vi "Format Error To Log Entry.vi"(6 "Error Call Chain":string[](array[string]), 7 "Event Level":T1, 8 "Error To Log":errorcluster, 9 "Event Time":timestamp, 10 "Error SourceID":string, 11 "Application Logger In":refnum<class "Application Logger.lvclass">) -> (2 "Log Packet":T2, 3 "Application Logger out":refnum<class "Application Logger.lvclass">)   [LabVIEW 2020, in "Composed Log.lvlib" / "Application Logger.lvclass"]
uses:
  <vilib>/gpm_packages/@cs/event-logger/Source/Composed Log/Application Logger/Application Logger.lvclass
  <vilib>/gpm_packages/@cs/event-logger/Source/Composed Log/Types/Log Packet.ctl
  <vilib>/gpm_packages/@cs/event-logger/Source/Composed Log/Types/Log Level.ctl
  <vilib>/gpm_packages/@cs/event-logger/Source/Composed Log/IErrorFormat/IErrorFormat.lvclass
  <vilib>/gpm_packages/@cs/event-logger/Source/Composed Log/Application Logger/Application Logger.lvclass/Application Logger.ctl
  <vilib>/gpm_packages/@cs/event-logger/Source/Composed Log/Composed Log.lvlib
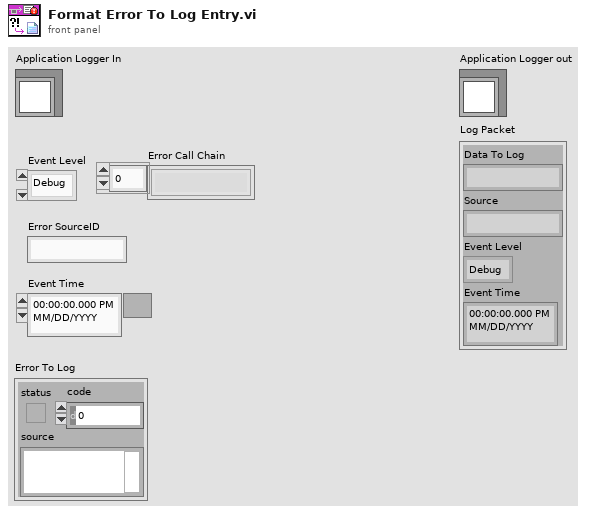
[diagram p1: front panel]
types:
  T1 = typedef "Composed Log.lvlib/Log Level.ctl" = enum16{"Debug", "Info", "Warning", "Error", "Critical"}
  T2 = typedef "Composed Log.lvlib/Log Packet.ctl" = cluster{"Data To Log":string, "Source":string, "Event Level":T1, "Event Time":timestamp}
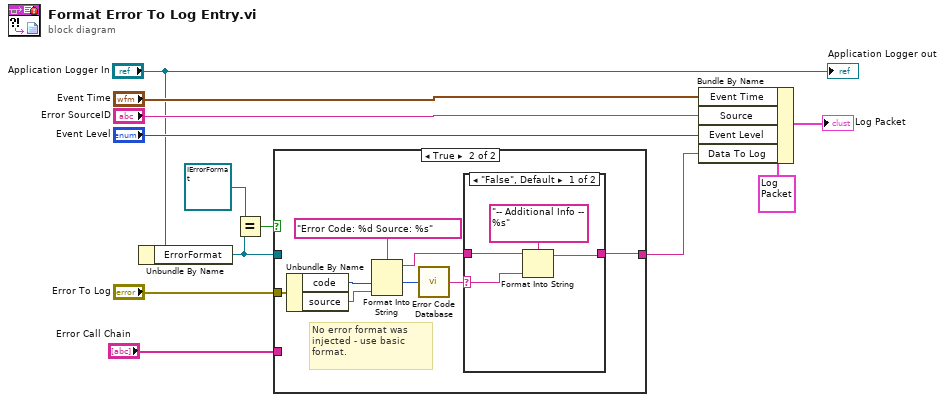
[diagram p0: block diagram]
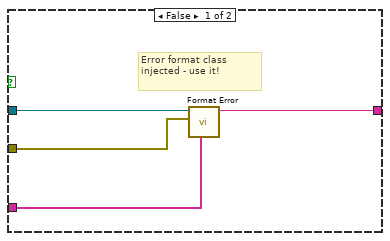
[diagram p2: hidden frame]
diagram:
  n1 = Unbundle By Name("Application Logger In") -> ("ErrorFormat"=w1:refnum<class "IErrorFormat.lvclass">)
  n2 = Equal?(x=refnum<class "IErrorFormat.lvclass"> refnum, y=w1) -> (x = y?=w2:bool)
  n3 = case shown="True" w2 {
    tunnel: "Error To Log" -> [w15 w23]
    tunnel: [w13 w17] -> w9
    tunnel: "Error Call Chain" -> [w14 _]
    tunnel: w1 -> [w16 _]
    frame False {
      # "Error format class injected - use it!"
      n4 = call-dynamic "Format Error.vi"("Call Chain"=w14, "Error To Log"=w15, "IErrorFormat in"=w16) -> ("Error String"=w13:string)  [unwired: 8 in]
    }
    frame True {
      # "No error format was injected - use basic format."
      n5 = Unbundle By Name(w23) -> ("code"=w21:i32, "source"=w20:string)
      n6 = Format Into String(format string="Error Code: %d Source: %s", w21, w20) -> (resulting string=w18:string)  [unwired: 2 in, 1 out]
      n7 = call <vilib>:"Error Code Database.vi"("Error Code"=w21) -> ("Error Text"=w19:string)
      n8 = case shown="\"False\", Default" w19 {
        selector: w19 -> [w25 _]
        tunnel: w18 -> [w27 w28]
        tunnel: [w24 w28] -> w17
        frame "False", Default {
          n9 = Format Into String(format string="-- Additional Info -- %s", initial string=w27, w25) -> (resulting string=w24:string)  [unwired: 1 in, 1 out]
        }
        frame "" {
        }
      }
    }
  }
  n10 = Bundle By Name(cluster=T2 {"Data To Log"="", "Source"="", "Event Level"=enum."Debug", "Event Time"=timestamp(0 s since 1904-01-01)} ("Log Packet"), "Event Time"="Event Time", "Source"="Error SourceID", "Event Level"="Event Level", "Data To Log"=w9) -> (→"Log Packet":T2)
  "Application Logger out" <- "Application Logger In"
